vi "Autocomplete UI.vi"(4 "LstBox Refnum":refnum<vi>, 5 "Ready Notifier":refnum<notifier>, 6 "Height (200)":i16=200, 7 "Stop Event":refnum<user-event>, 8 "Options":refnum<user-event>, 11 "Str Refnum":refnum<vi>) -> ()   [LabVIEW 2020, in "FlexBlocks.lvlib"]
uses:
  FlexBlocks.lvlib
  <vilib>/Utility/miscctls.llb/LVRectTypeDef.ctl
  <vilib>/event_ctls.llb/eventvkey.ctl
panel:
  out "All Options":string[](array[string])
  in  "Listbox":i32(listbox)
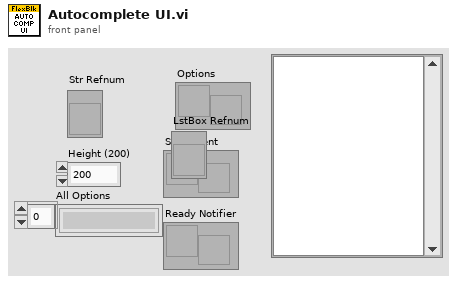
[diagram p1: front panel]
types:
  T1 = typedef "LVRectTypeDef.ctl" = cluster{"Left":i16, "Top":i16, "Right":i16, "Bottom":i16}
  T2 = enum32{"Invalid", "Standard", "Closed", "Hidden", "Minimized", "Maximized"}
  T3 = typedef "eventvkey.ctl" = enum16{"ASCII", "Enter", "Return", "Shift", "Ctrl", "Alt", "Cmd", "Opt", "Caps", "NumLock", "Clear", "Break", "Up", "Down", "Left", "Right", "Insert", "Delete", "Home", "End", "PageUp", "PageDown", "Escape", "Help", "Pause", "ScrollLock", "F1", "F2", "F3", "F4", "F5", "F6", "F7", "F8", "F9", "F10", "F11", "F12", "F13", "F14", "F15", "F16", "F17", "F18", "F19", "F20", "F21", "F22", "F23", "F24", "Play", "VolumeUp", "VolumeDown", "Mute", "Two Byte Char"}
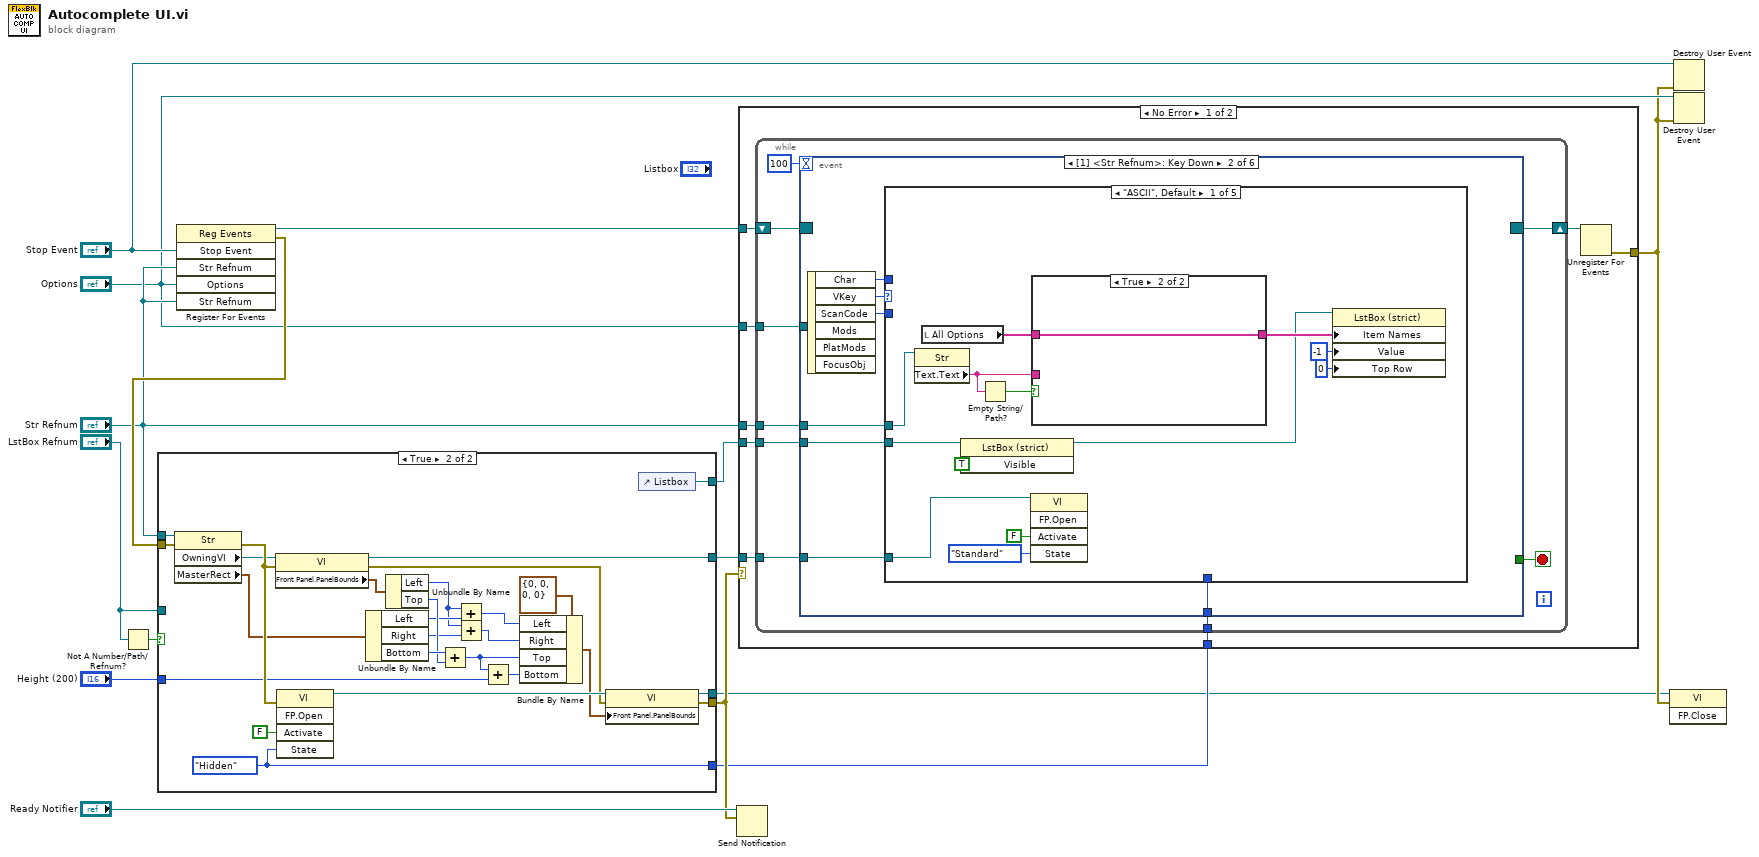
[diagram p0: block diagram]
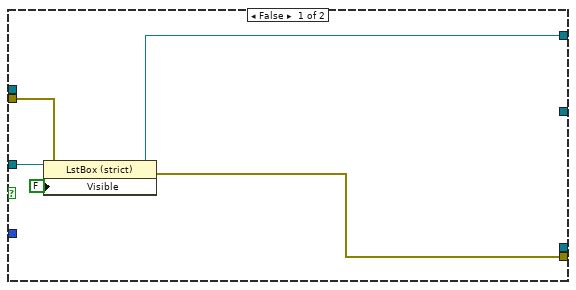
[diagram p2: hidden frame]
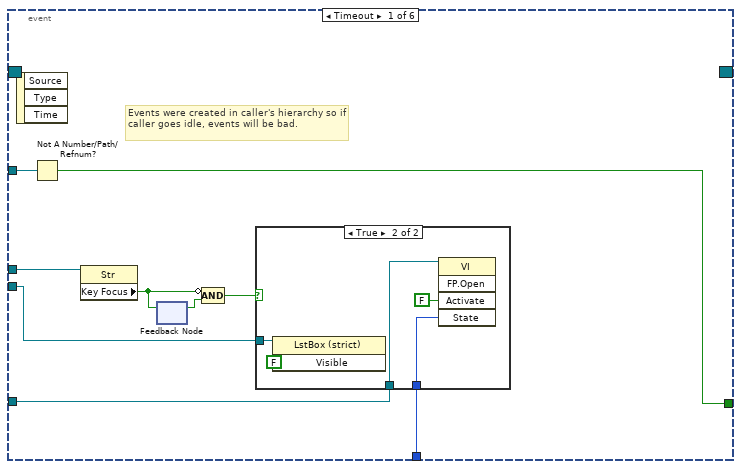
[diagram p3: hidden frame]
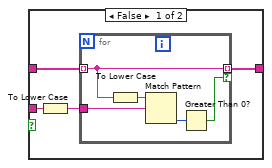
[diagram p5: hidden frame]
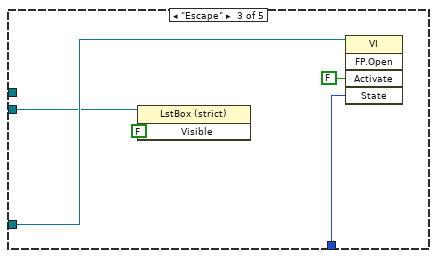
[diagram p7: hidden frame]
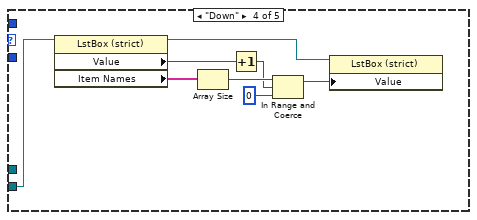
[diagram p8: hidden frame]
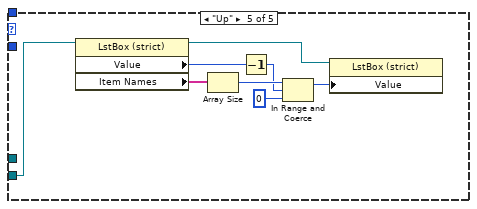
[diagram p9: hidden frame]
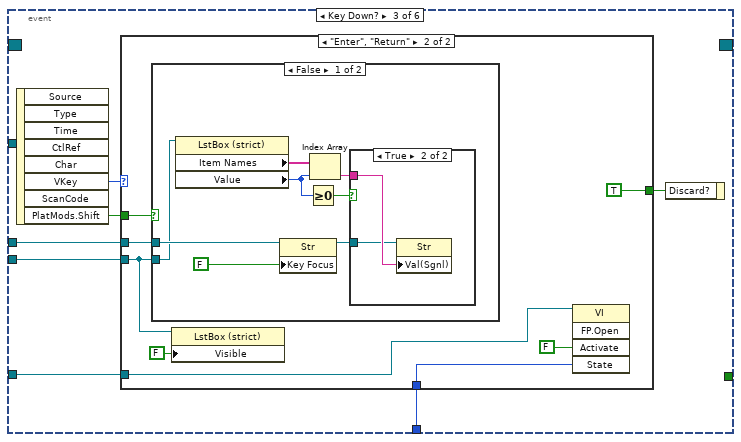
[diagram p10: hidden frame]
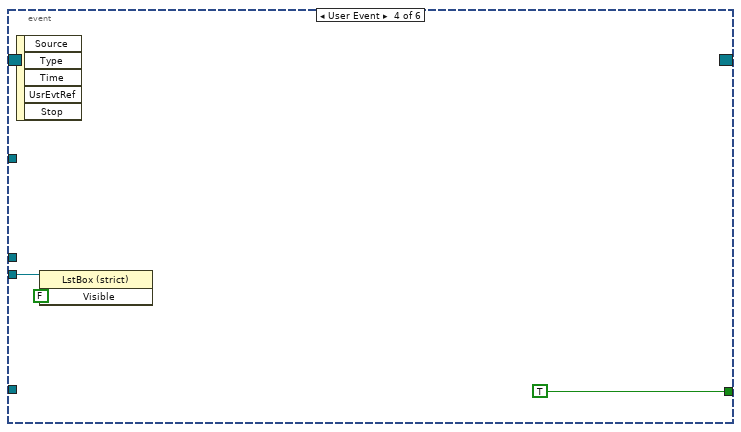
[diagram p14: hidden frame]
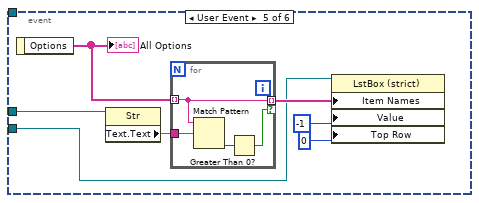
[diagram p15: hidden frame]
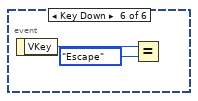
[diagram p16: hidden frame]
diagram:
  n1 = Not A Number/Path/Refnum?(number/path/refnum="LstBox Refnum") -> (NaN/Path/Refnum?=w3:bool)
  n2 = register-events("Stop Event", "Str Refnum", "Options", "Str Refnum") -> (reference out=w14:refnum<event-registration>, error out=w15:errorcluster)  [unwired: 2 in]
  n3 = case shown="True" w3 {
    tunnel: w15 -> [w18 w46]
    tunnel: "Height (200)" -> [_ w42]
    tunnel: [_ w38] -> w12
    tunnel: [w17 w37] -> w10
    tunnel: "Str Refnum" -> [_ w36]
    tunnel: [_ w23] -> w6
    tunnel: [_ w22] -> w4
    tunnel: "LstBox Refnum" -> [w20 _]
    tunnel: [w16 w21] -> w1
    frame False {
      n4 = property class="LstBox (strict)"(reference=w20, error in=w18, "Visible"=FALSE) -> (reference out=w16:refnum<vi>, error out=w17:errorcluster)
    }
    frame True {
      w23 = T2."Hidden" ("State")
      n5 = property class="Str"(reference=w36, error in=w46) -> (error out=w45:errorcluster, "OwningVI"=w39:refnum<vi>, "MasterRect"=w35:T1)  [unwired: 1 out]
      n6 = property class="VI"(reference=w39, error in=w45) -> (reference out=w38:refnum<vi>, error out=w40:errorcluster, "Front Panel.PanelBounds"=w34:T1)
      n7 = invoke class="VI" method="FP.Open"(error in=w45, "Activate"=FALSE ("Activate?"), "State"=w23) -> (reference out=w43:refnum<vi>)  [unwired: 2 in, 4 out]
      n8 = Unbundle By Name(w35) -> ("Left"=w29:i16, "Right"=w30:i16, "Bottom"=w33:i16)
      n9 = Unbundle By Name(w34) -> ("Left"=w28:i16, "Top"=w31:i16)
      n10 = Add(x=w33, y=w31) -> (x+y=w32:i16)
      n11 = Add(x=w28, y=w29) -> (x+y=w24:i16)
      n12 = Add(x=w28, y=w30) -> (x+y=w25:i16)
      n13 = Add(x=w32, y=w42) -> (x+y=w41:i16)
      n14 = Bundle By Name(cluster=T1 {"Left"=0, "Top"=0, "Right"=0, "Bottom"=0} ("Front Panel Window:Panel Bounds"), "Left"=w24, "Right"=w25, "Top"=w32, "Bottom"=w41) -> (w27:T1)
      n15 = property class="VI"(reference=w43, error in=w40, "Front Panel.PanelBounds"=w27) -> (reference out=w22:refnum<vi>, error out=w37:errorcluster)
      n16 = control-ref of="Listbox"() -> (w21:refnum<vi>)
    }
  }
  n17 = Send Notification(notification=w10, notifier="Ready Notifier") -> ()  [unwired: 1 in, 2 out]
  n18 = case shown="No Error" w10 {
    tunnel: w14 -> [w54 _]
    tunnel: "Str Refnum" -> [w53 _]
    tunnel: [w51 _] -> w5
    tunnel: w12 -> [w50 _]
    tunnel: "Options" -> [w49 _]
    tunnel: w6 -> [w48 _]
    tunnel: w1 -> [w47 _]
    frame No Error {
      n19 = while {
        shift-right: [w62] -> w52
        shift-left: w54 -> [w63]
        tunnel: w53 -> [w60]
        tunnel: w50 -> [w58]
        tunnel: w49 -> [w57]
        tunnel: w48 -> [w56]
        tunnel: w47 -> [w55]
        stop <- w61 stop-if-true
        n20 = event shown="[1] <Str Refnum>: Key Down" {
          selector: w63 -> [_ _ _ _ _ _]
          dyn-events: [_ _ _ _ _ _] -> w62
          timeout: 100 -> [_ _ _ _ _ _]
          tunnel: [w67 _ _ TRUE _ _] -> w61
          tunnel: w60 -> [w72 w83 w132 _ w158 _]
          tunnel: w58 -> [w65 w79 w130 _ _ _]
          tunnel: w57 -> [w68 _ _ _ _ _]
          tunnel: w56 -> [w66 w80 w131 _ _ _]
          tunnel: w55 -> [w64 w78 w129 w155 w157 _]
          event Timeout {
            # "Events were created in caller's hierarchy so if caller goes idle, events will be bad."
            n21 = event-data() -> ()  [unwired: 1 in, 3 out]
            n22 = Not A Number/Path/Refnum?(number/path/refnum=w68) -> (NaN/Path/Refnum?=w67:bool)
            n23 = property class="Str"(reference=w72) -> ("Key Focus"=w71:bool)  [unwired: 1 in, 2 out]
            n24 = feedback-in #1(w71) -> ()
            n25 = feedback #1() -> (w70:bool)  [unwired: 1 in]
            n26 = Compound Arithmetic op=AND(invert w71, w70) -> (w69:bool)
            n27 = case shown="True" w69 {
              tunnel: w66 -> [_ w76]
              tunnel: w65 -> [_ w75]
              tunnel: w64 -> [_ w73]
              frame False {
              }
              frame True {
                n28 = property class="LstBox (strict)"(reference=w73, "Visible"=FALSE) -> ()  [unwired: 1 in, 2 out]
                n29 = invoke class="VI" method="FP.Open"(reference=w75, "Activate"=FALSE ("Activate?"), "State"=w76) -> ()  [unwired: 2 in, 5 out]
              }
            }
          }
          event Key Down {
            n30 = event-data() -> ("Char"=w82:i16, "VKey"=w84:T3, "ScanCode"=w81:i16)  [unwired: 1 in, 3 out]
            n31 = case shown="\"ASCII\", Default" w84 {
              tunnel: w83 -> [w96 _ _ _ _]
              tunnel: w82 -> [_ _ _ _ _]
              tunnel: w81 -> [_ _ _ _ _]
              tunnel: w80 -> [_ _ w111 _ _]
              tunnel: w79 -> [w90 _ w110 _ _]
              tunnel: w78 -> [w89 _ w109 w114 w121]
              frame "ASCII", Default {
                n32 = property class="Str"(reference=w96) -> ("Text.Text"=w86:string)  [unwired: 1 in, 2 out]
                n33 = local read "All Options"() -> (w91:string[])
                n34 = property class="LstBox (strict)"(reference=w89, "Visible"=TRUE) -> (reference out=w87:refnum<vi>)  [unwired: 1 in, 1 out]
                n35 = Empty String/Path?(string/path=w86) -> (empty?=w85:bool)
                n36 = invoke class="VI" method="FP.Open"(reference=w90, "Activate"=FALSE ("Activate?"), "State"=T2."Standard") -> ()  [unwired: 2 in, 5 out]
                n37 = case shown="True" w85 {
                  tunnel: [w101 w107] -> w92
                  tunnel: w91 -> [w100 w107]
                  tunnel: w86 -> [w98 _]
                  frame False {
                    n38 = To Lower Case(string=w98) -> (all lower case string=w99:string)
                    n39 = for {
                      tunnel: w99 -> [w104]
                      tunnel: [w103] -> w101 mode=indexing if=w105
                      tunnel: w100 -> [w103] mode=indexing
                      n40 = To Lower Case(string=w103) -> (all lower case string=w102:string)
                      n41 = Match Pattern(string=w102, regular expression=w104) -> (offset past match=w106:i32)  [unwired: 1 in, 3 out]
                      n42 = Greater Than 0?(x=w106) -> (x > 0?=w105:bool)
                    }
                  }
                  frame True {
                  }
                }
                n43 = property on="Property Node" class="LstBox (strict)"(reference=w87, "Item Names"=w92, "Value"=-1 ("Listbox"), "Top Row"=0) -> ()  [unwired: 1 in, 2 out]
              }
              frame "Enter", "Return" {
                # "Handled in Key Down?"
              }
              frame "Escape" {
                n44 = property class="LstBox (strict)"(reference=w109, "Visible"=FALSE) -> ()  [unwired: 1 in, 2 out]
                n45 = invoke class="VI" method="FP.Open"(reference=w110, "Activate"=FALSE ("Activate?"), "State"=w111) -> ()  [unwired: 2 in, 5 out]
              }
              frame "Down" {
                n46 = property on="Property Node" class="LstBox (strict)"(reference=w114) -> (reference out=w113:refnum<vi>, "Value"=w119:i32, "Item Names"=w120:string[])  [unwired: 1 in, 1 out]
                n47 = Array Size(array=w120) -> (size(s)=w118:i32)
                n48 = Increment(x=w119) -> (x+1=w117:i32)
                n49 = In Range and Coerce(upper limit=w118, x=w117, lower limit=0) -> (coerced(x)=w115:i32)  [unwired: 1 out]
                n50 = property on="Property Node" class="LstBox (strict)"(reference=w113, "Value"=w115) -> ()  [unwired: 1 in, 2 out]
              }
              frame "Up" {
                n51 = property on="Property Node" class="LstBox (strict)"(reference=w121) -> (reference out=w122:refnum<vi>, "Value"=w127:i32, "Item Names"=w128:string[])  [unwired: 1 in, 1 out]
                n52 = Array Size(array=w128) -> (size(s)=w126:i32)
                n53 = Decrement(x=w127) -> (x-1=w125:i32)
                n54 = In Range and Coerce(upper limit=w126, x=w125, lower limit=0) -> (coerced(x)=w123:i32)  [unwired: 1 out]
                n55 = property on="Property Node" class="LstBox (strict)"(reference=w122, "Value"=w123) -> ()  [unwired: 1 in, 2 out]
              }
            }
          }
          event Key Down? {
            n56 = event-data() -> ("VKey"=w135:T3, "PlatMods.Shift"=w134:bool)  [unwired: 1 in, 6 out]
            n57 = case shown="\"Enter\", \"Return\"" w135 {
              tunnel: w134 -> [_ w143]
              tunnel: [_ TRUE] -> w133
              tunnel: w132 -> [_ w140]
              tunnel: w131 -> [_ w139]
              tunnel: w130 -> [_ w138]
              tunnel: w129 -> [_ w136]
              frame "ASCII", Default {
              }
              frame "Enter", "Return" {
                n58 = case shown="False" w143 {
                  tunnel: w140 -> [w146 _]
                  tunnel: w136 -> [w144 _]
                  frame False {
                    n59 = property on="Property Node" class="LstBox (strict)"(reference=w144) -> ("Item Names"=w151:string[], "Value"=w150:i32)  [unwired: 1 in, 2 out]
                    n60 = property class="Str"(reference=w146, "Key Focus"=FALSE) -> (reference out=w145:refnum<vi>)  [unwired: 1 in, 1 out]
                    n61 = Greater Or Equal To 0?(x=w150) -> (x >= 0?=w149:bool)
                    n62 = Index Array(array=w151, index=w150) -> (element=w148:string)
                    n63 = case shown="True" w149 {
                      tunnel: w148 -> [_ w153]
                      tunnel: w145 -> [_ w152]
                      frame False {
                      }
                      frame True {
                        n64 = property class="Str"(reference=w152, "Val(Sgnl)"=w153) -> ()  [unwired: 1 in, 2 out]
                      }
                    }
                  }
                  frame True {
                  }
                }
                n65 = property class="LstBox (strict)"(reference=w136, "Visible"=FALSE) -> ()  [unwired: 1 in, 2 out]
                n66 = invoke class="VI" method="FP.Open"(reference=w138, "Activate"=FALSE ("Activate?"), "State"=w139) -> ()  [unwired: 2 in, 5 out]
              }
            }
            n67 = event-data("Discard?"=w133) -> ()  [unwired: 1 in, 1 out]
          }
          event User Event {
            n68 = event-data() -> ()  [unwired: 1 in, 5 out]
            n69 = property class="LstBox (strict)"(reference=w155, "Visible"=FALSE) -> ()  [unwired: 1 in, 2 out]
          }
          event User Event {
            n70 = event-data() -> ("Options"=w159:string[])  [unwired: 1 in]
            "All Options" <- w159
            n71 = property class="Str"(reference=w158) -> ("Text.Text"=w162:string)  [unwired: 1 in, 2 out]
            n72 = for {
              tunnel: w162 -> [w165]
              tunnel: [w164] -> w160 mode=indexing if=w166
              tunnel: w159 -> [w164] mode=indexing
              n73 = Match Pattern(string=w164, regular expression=w165) -> (offset past match=w167:i32)  [unwired: 1 in, 3 out]
              n74 = Greater Than 0?(x=w167) -> (x > 0?=w166:bool)
            }
            n75 = property on="Property Node" class="LstBox (strict)"(reference=w157, "Item Names"=w160, "Value"=-1 ("Listbox"), "Top Row"=0) -> ()  [unwired: 1 in, 2 out]
          }
          event Key Down {
            n76 = event-data() -> ("VKey"=w169:T3)  [unwired: 1 in]
            n77 = Equal?(x=w169, y=eventvkey."Escape") -> ()  [unwired: 1 out]
          }
        }
      }
      n78 = Unregister For Events(event registration refnum=w52) -> (error out=w51:errorcluster)  [unwired: 1 in]
    }
    frame Error {
    }
  }
  n79 = invoke class="VI" method="FP.Close"(reference=w4, error in=w5) -> ()  [unwired: 1 in, 3 out]
  n80 = Destroy User Event(user event="Stop Event", error in=w5) -> ()  [unwired: 1 out]
  n81 = Destroy User Event(user event="Options", error in=w5) -> ()  [unwired: 1 out]
